vi "Scope Channel UI.vi"() -> ()   [LabVIEW 2025, in "Scope.lvlib" / "Scope Channel.lvclass"]
doc: "Tab Control"
uses:
  Scope Channel.lvclass
  Users/Public/Documents/Sandia National Labs/TSS Plugin/CEF.lvlibp/Node/NodeRef.ctl
  Users/Public/Documents/Sandia National Labs/TSS Plugin/CEF.lvlibp/Node/CEF_Node.lvclass
  Users/Public/Documents/Sandia National Labs/TSS Plugin/CEF.lvlibp/Node/mainQref.ctl
  Users/Public/Documents/Sandia National Labs/TSS Plugin/CEF.lvlibp/Node/UserEventRef.ctl
  Users/Public/Documents/Sandia National Labs/TSS Plugin/Abstract Engine.lvlibp/Plugin/Abstract/Channel configuration/Default Channel.ctl
  Scope Channel configuration/Scope Channel Setting.ctl
  C:/Users/Public/Documents/Sandia National Labs/TSS Plugin/CEF.lvlibp/Node/CEF_Node.lvclass
  Scope Channel.lvclass/Scope Channel.ctl
  Scope Channel configuration/Scope Channel configuration.lvclass/Scope Channel configuration.ctl
  Scope Channel configuration/Read Scope Channel.vi
  Scope Channel configuration/Write Scope Channel.vi
  <vilib>/Utility/error.llb/Trim Whitespace One-Sided.vi
  Scope Channel configuration/Scope Channel configuration.lvclass
  C:/Users/Public/Documents/Sandia National Labs/TSS Plugin/Abstract Engine.lvlibp/Plugin/Abstract/Channel configuration/Channel configuration.lvclass
  Users/Public/Documents/Sandia National Labs/TSS Plugin/Abstract Engine.lvlibp/Plugin/Abstract/Channel configuration/Read Channel Setting.vi
  Users/Public/Documents/Sandia National Labs/TSS Plugin/Abstract Engine.lvlibp/Plugin/Abstract/Channel configuration/Write Channel Setting.vi
  Users/Public/Documents/Sandia National Labs/TSS Plugin/Abstract Engine.lvlibp/Plugin/Abstract/Channel configuration/Channel configuration.lvclass
panel:
  in  "Scope Channel":cluster{"Default":T1, "Setting":T2}={"Default"={"Address"="None", "SW Alias"="0", "Enabled"=TRUE, "Type"="Scope Channel", "Description"="* Type = Channel Class"}, "Setting"={"Gain"=1, "Offset"=0, "Vertical Range"=10.0, "Vertical Offset"=0.0, "Unit"="V", "Attenuation"=1.0, "Vertical Coupling"="DC", "Impedance"="1M", "Auto Setup"=TRUE}}
  in  "user event":T3
  in  "main queue":T4
  in  "node ref":T5
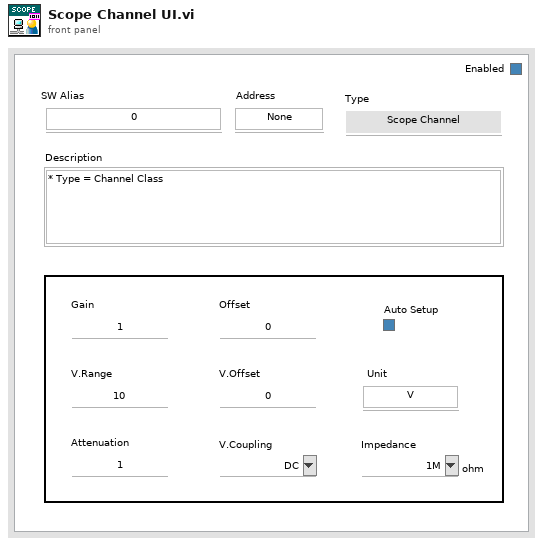
[diagram p1: front panel]
types:
  T1 = typedef "Abstract Engine.lvlibp/Channel configuration.lvclass/Default Channel.ctl" = cluster{"Address":string, "SW Alias":string, "Enabled":bool, "Type":string, "Description":string}
  T2 = typedef "Scope.lvlib/Scope Channel configuration.lvclass/Scope Channel Setting.ctl" = cluster{"Gain":u32, "Offset":u32, "Vertical Range":dbl, "Vertical Offset":dbl, "Unit":string, "Attenuation":dbl, "Vertical Coupling":string, "Impedance":string, "Auto Setup":bool}
  T3 = typedef "CEF.lvlibp/CEF_Node.lvclass/UserEventRef.ctl" = refnum<user-event>
  T4 = typedef "CEF.lvlibp/CEF_Node.lvclass/mainQref.ctl" = refnum<queue>
  T5 = typedef "CEF.lvlibp/CEF_Node.lvclass/NodeRef.ctl" = refnum<data-value>
  T6 = cluster{"Channel Setting":T1, "Scope Channel":T2}
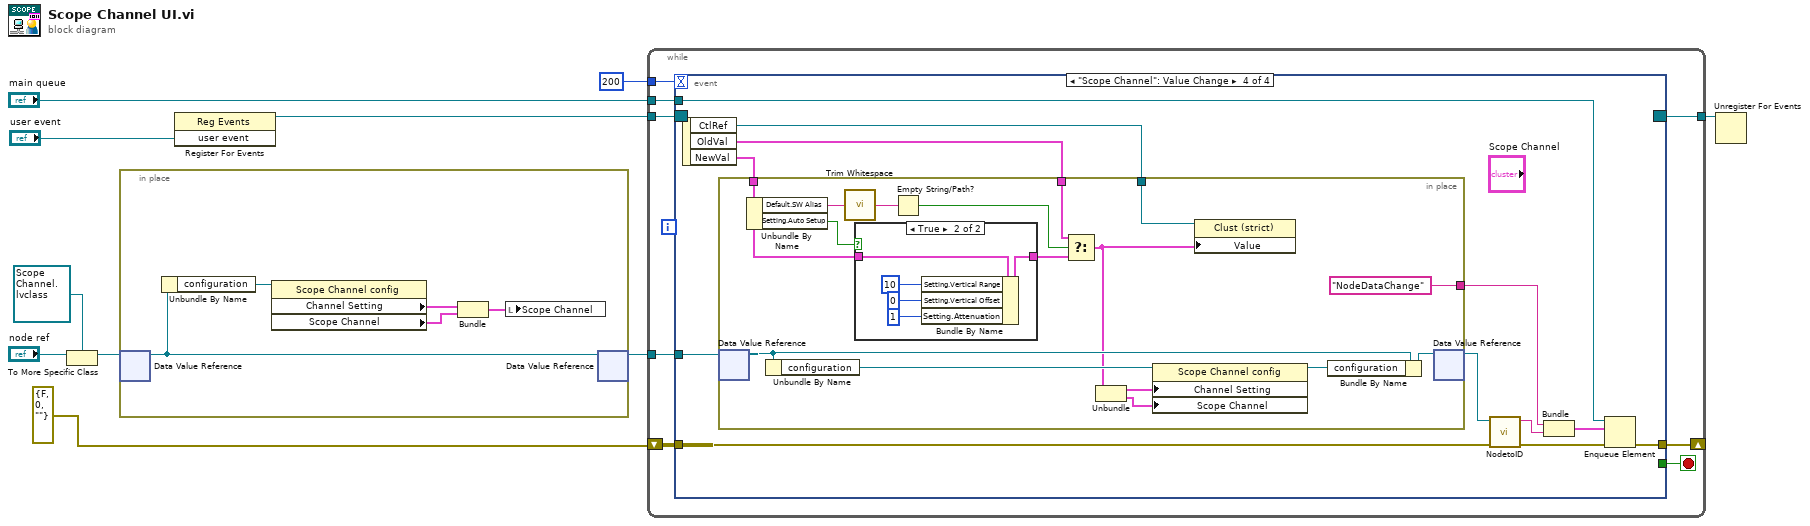
[diagram p0: block diagram]
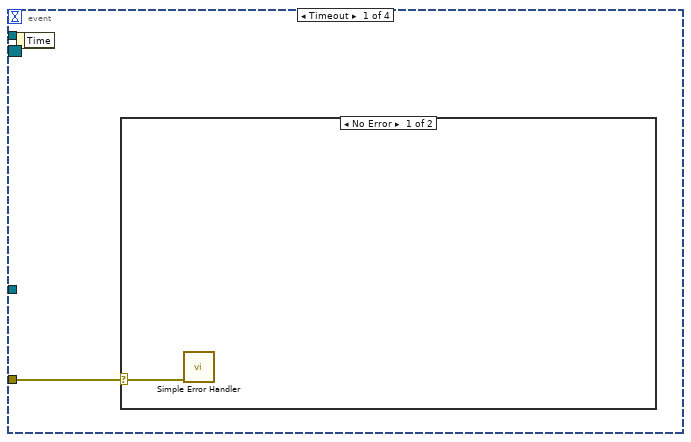
[diagram p2: hidden frame]
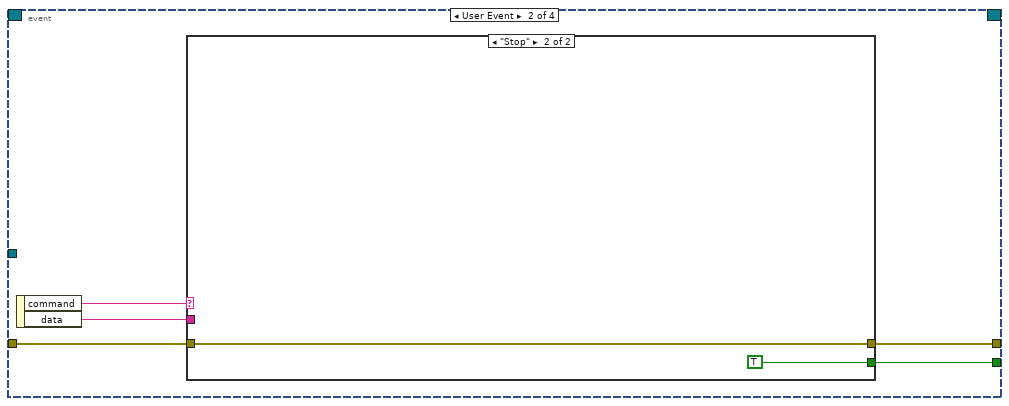
[diagram p4: hidden frame]
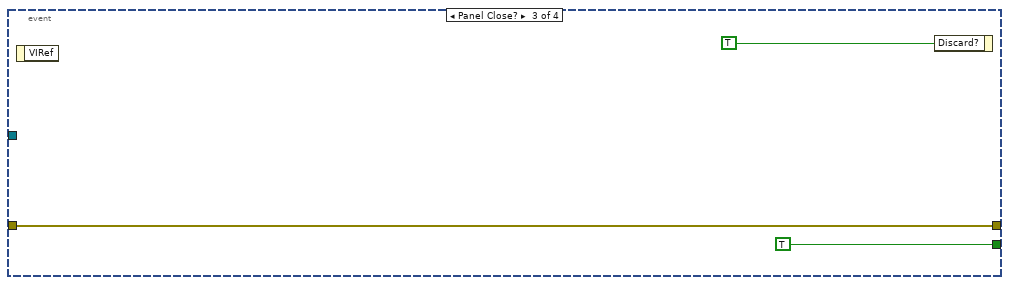
[diagram p6: hidden frame]
diagram:
  n1 = To More Specific Class(target class=refnum<data-value> refnum ("data value reference"), reference="node ref") -> (specific class reference=w3:refnum<data-value>)  [unwired: 1 in, 1 out]
  n2 = in-place {
    # "Initialize the front panel controls when loaded"
    n3 = in-place-dvr #1(w3) -> (w15:refnum<class "Scope Channel.lvclass">)  [unwired: 1 out]
    n4 = Unbundle By Name(w15) -> ("configuration"=w14:refnum<class "Scope Channel configuration.lvclass">)
    n5 = property class="Scope Channel config"(reference=w14) -> ("Channel Setting"=w13:T1, "Scope Channel"=w12:T2)  [unwired: 1 in, 2 out]
    n6 = Bundle("Channel Setting"=w13, "Scope Channel"=w12) -> (w11:T6)  [unwired: 1 in]
    n7 = local write "Scope Channel"(w11) -> ()
    n8 = in-place-dvr #1(w15) -> (w4:refnum<data-value>)  [unwired: 1 out]
  }
  n9 = register-events("user event") -> (reference out=w9:refnum<event-registration>)  [unwired: 2 in, 1 out]
  n10 = while {
    tunnel: w4 -> [w23]
    tunnel: w9 -> [w22]
    tunnel: [w21] -> w8
    tunnel: "main queue" -> [w18]
    tunnel: 200 -> [w16]
    shift-right: [w19] -> _
    shift-left: errorcluster {"status"=FALSE, "code"=0, "source"=""} ("error out") -> [w17]
    stop <- w20 stop-if-true
    n11 = event shown="[3] \"Scope Channel\": Value Change" {
      selector: w22 -> [_ _ _ _]
      dyn-events: [_ _ _ _] -> w21
      timeout: w16 -> [_ _ _ _]
      tunnel: w23 -> [_ _ _ w46]
      tunnel: [_ w30 TRUE _] -> w20
      tunnel: [_ w26 w34 w47] -> w19
      tunnel: w18 -> [_ _ _ w48]
      tunnel: w17 -> [w24 w27 w34 w37]
      event Timeout {
        n12 = event-data() -> ()  [unwired: 1 in, 1 out]
        n13 = case shown="No Error" w24 {
          selector: w24 -> [w25 _]
          frame No Error {
            n14 = call <vilib>:"Simple Error Handler.vi"("error in (no error)"=w25) -> ()  [unwired: 4 in, 5 out]
          }
          frame Error {
          }
        }
      }
      event User Event {
        n15 = event-data() -> ("command"=w29:string, "data"=w28:string)  [unwired: 1 in]
        n16 = case shown="\"Stop\"" w29 {
          tunnel: w28 -> [_ _]
          tunnel: [_ TRUE] -> w30
          tunnel: w27 -> [w31 w32]
          tunnel: [w31 w32] -> w26
          frame Default {
          }
          frame "Stop" {
          }
        }
      }
      event Panel Close? {
        n17 = event-data() -> ()  [unwired: 1 in, 1 out]
        n18 = event-data("Discard?"=TRUE ("Run")) -> ()  [unwired: 1 in, 1 out]
      }
      event "Scope Channel": Value Change {
        n19 = event-data() -> ("CtlRef"=w42:refnum<vi>, "OldVal"=w43:cluster{"Default":T1, "Setting":T2}, "NewVal"=w44:cluster{"Default":T1, "Setting":T2})  [unwired: 1 in]
        n20 = in-place {
          in-place-border: w44 -> [w57]
          in-place-border: w43 -> [w56]
          in-place-border: w42 -> [w55]
          in-place-border: ["NodeDataChange" ("Message Name")] -> w41
          n21 = in-place-dvr #2(w46) -> (w64:refnum<class "Scope Channel.lvclass">)  [unwired: 1 out]
          n22 = Unbundle By Name(w57) -> ("Default.SW Alias"=w60:string, "Setting.Auto Setup"=w51:bool)
          n23 = Unbundle By Name(w64) -> ("configuration"=w62:refnum<class "Scope Channel configuration.lvclass">)
          n24 = call <vilib>:"Trim Whitespace.vi"("string"=w60) -> ("trimmed string"=w54:string)  [unwired: 1 in]
          n25 = case shown="True" w51 {
            tunnel: w57 -> [w65 w70]
            tunnel: [w65 w66] -> w58
            frame False {
            }
            frame True {
              n26 = Bundle By Name(cluster=w70, "Setting.Vertical Range"=u32 10, "Setting.Vertical Offset"=u32 0, "Setting.Attenuation"=u32 1 ("Setting.Probe Attenuation")) -> (w66:cluster{"Default":T1, "Setting":T2})
            }
          }
          n27 = Empty String/Path?(string/path=w54) -> (empty?=w59:bool)
          n28 = Select(t=w56, s=w59, f=w58) -> (s? t:f=w53:cluster{"Default":T1, "Setting":T2})
          n29 = Unbundle(w53) -> ("Default"=w49:T1, "Setting"=w52:T2)
          n30 = property class="Scope Channel config"(reference=w62, "Channel Setting"=w49, "Scope Channel"=w52) -> (reference out=w61:refnum<class "Scope Channel configuration.lvclass">)  [unwired: 1 in, 1 out]
          n31 = property class="Clust (strict)"(reference=w55, "Value"=w53) -> ()  [unwired: 1 in, 2 out]
          n32 = Bundle By Name(cluster=w64, "configuration"=w61) -> (w63:refnum<class "Scope Channel.lvclass">)
          n33 = in-place-dvr #2(w63) -> (w45:refnum<data-value>)  [unwired: 1 out]
        }
        n34 = call "NodetoID.vi"("error in"=w37, "node ref"=w45) -> ("error out"=w38:errorcluster, "ID"=w40:string)  [unwired: 8 in]
        n35 = Bundle("Message Name"=w41, "ID"=w40) -> (w39:cluster{"Message Name":string, "ID":string})  [unwired: 1 in]
        n36 = Enqueue Element(queue=w48, element=w39, error in (no error)=w38) -> (error out=w47:errorcluster)  [unwired: 1 in, 2 out]
      }
    }
  }
  n37 = Unregister For Events(event registration refnum=w8) -> ()  [unwired: 1 in, 1 out]
